vi "Bloch Sphere - Display.vi"(7 "QuWire in":refnum<class "QuWire.lvclass">) -> ()   [LabVIEW 2020]
uses:
  QuSim/QuWire/QuWire.lvclass
  <vilib>/Utility/miscctls.llb/LV3DPointTypeDef.ctl
  <vilib>/picture/3D Picture Control/NI_3D Picture Control.lvlib
panel:
  out "3D Picture":refnum<vi>(3d-picture)
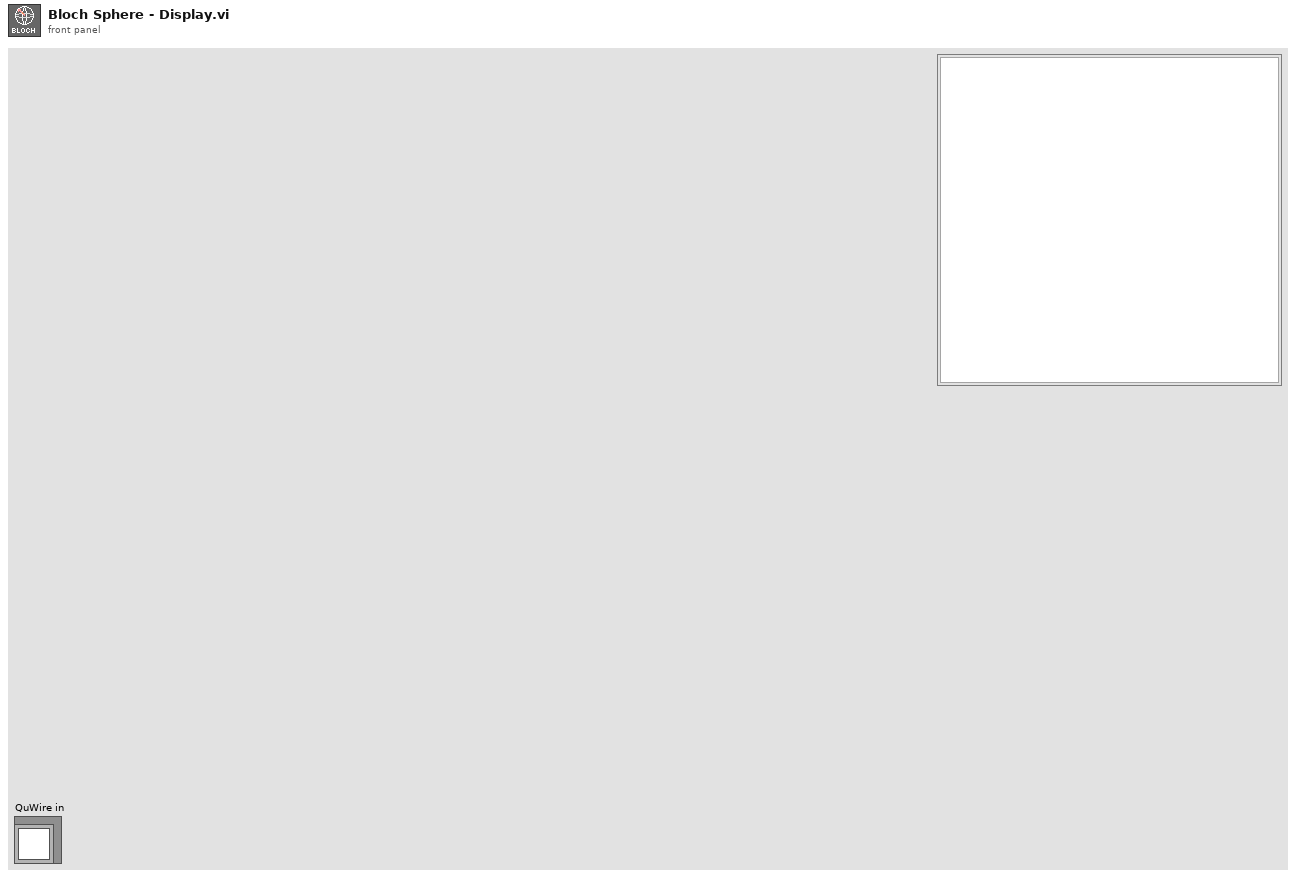
[diagram p1: front panel]
types:
  T1 = typedef "LV3DPointTypeDef.ctl" = cluster{"X":sgl, "Y":sgl, "Z":sgl}
  T2 = enum16{"None", "Spherical", "Flying", "Oriented"}
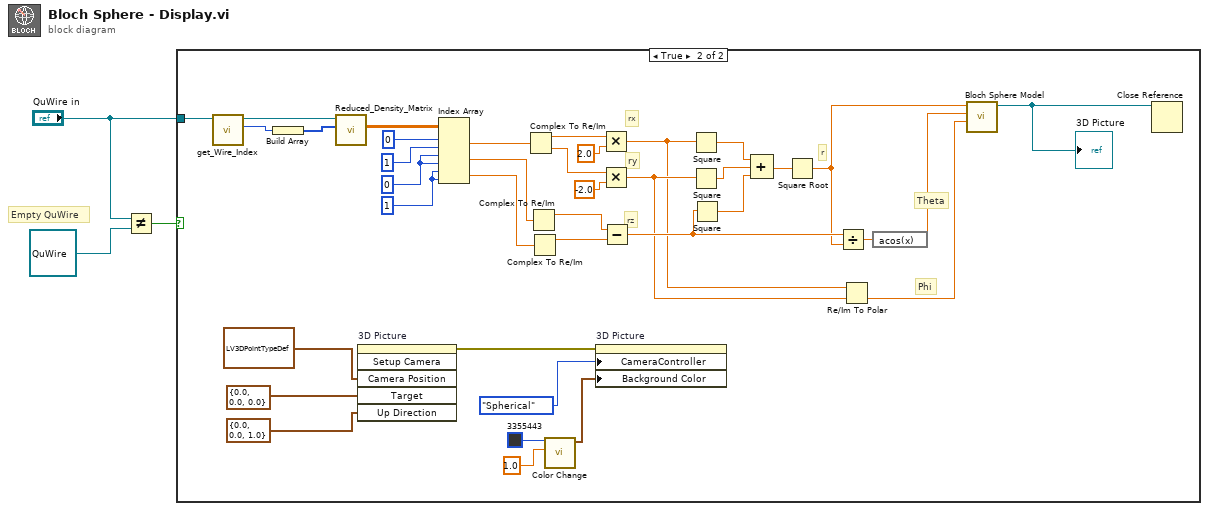
[diagram p0: block diagram]
diagram:
  # "Empty QuWire"
  n1 = Not Equal?(x="QuWire in", y=refnum<class "QuWire.lvclass"> refnum ("QuWire in")) -> (x != y?=w2:bool)
  n2 = case shown="True" w2 {
    tunnel: "QuWire in" -> [_ w18]
    frame False {
    }
    frame True {
      w38 = 1 ("disabled index (col)")
      w39 = 0 ("index (row)")
      # "Phi"
      # "Theta"
      # "r"
      # "rz"
      # "ry"
      # "rx"
      n3 = call "get_Wire_Index.vi"("QuWire in"=w18) -> ("Wire Index"=w16:i32, "QuWire out"=w17:refnum<class "QuWire.lvclass">)  [unwired: 8 in, 1 out]
      n4 = Build Array(w16) -> (w20:i32[])
      n5 = call "Reduced_Density_Matrix.vi"("Qubits to Keep"=w20, "QuWire in"=w17) -> ("Reduced Density Matrix"=w19:cdb[][])  [unwired: 6 in, 3 out]
      n6 = invoke on="3D Picture" class="SceneGraphDisp (strict)" method="Setup Camera"("Camera Position"=T1 {"X"=2.4, "Y"=1.6, "Z"=1.6}, "Target"=T1 {"X"=0.0, "Y"=0.0, "Z"=0.0}, "Up Direction"=T1 {"X"=0.0, "Y"=0.0, "Z"=1.0}) -> (error out=w8:errorcluster)  [unwired: 3 in, 5 out]
      n7 = Index Array(array=w19, index (row) #1=0 ("index (row)"), index (col) #1=1 ("disabled index (col)"), index (row) #2=w39, index (col) #2=w39, index (row) #3=w38, index (col) #3=w38) -> (element #1=w37:cdb, element #2=w31:cdb, element #3=w30:cdb)
      n8 = Complex To Re/Im(x + iy=w37) -> (x=w36:dbl, y=w33:dbl)
      n9 = Complex To Re/Im(x + iy=w31) -> (x=w28:dbl)  [unwired: 1 out]
      n10 = Complex To Re/Im(x + iy=w30) -> (x=w29:dbl)  [unwired: 1 out]
      n11 = call <vilib>:"Color Change.vi"("Alpha"=1.0, "Color"=u32 3355443 ("BG Color")) -> ("RGBA"=w7:cluster{"R":sgl, "G":sgl, "B":sgl, "A":sgl})  [unwired: 9 in]
      n12 = property on="3D Picture" class="SceneGraphDisp (strict)"(error in=w8, "CameraController"=T2."Spherical" ("Camera Controller:Type"), "Background Color"=w7) -> ()  [unwired: 1 in, 2 out]
      n13 = Multiply(x=w36, y=2.0) -> (x*y=w21:dbl)
      n14 = Multiply(x=w33, y=-2.0) -> (x*y=w22:dbl)
      n15 = Subtract(x=w28, y=w29) -> (x-y=w26:dbl)
      n16 = Square(x=w21) -> (x^2=w24:dbl)
      n17 = Square(x=w22) -> (x^2=w23:dbl)
      n18 = Square(x=w26) -> (x^2=w32:dbl)
      n19 = Compound Arithmetic op=ADD(w24, w23, w32) -> (w27:dbl)
      n20 = Square Root(x=w27) -> (sqrt(x)=w14:dbl)
      n21 = Divide(x=w26, y=w14) -> (x/y=w25:dbl)
      n22 = Re/Im To Polar(2:w22, 3:w21) -> (0:w12:dbl)  [unwired: 1 out]
      n23 = expression code="acos(x)"(w25) -> (w13:dbl)
      n24 = call "Bloch Sphere Model.vi"("Phi"=w12, "Theta"=w13, "Length"=w14) -> ("SceneObject out"=w15:refnum<vi>)  [unwired: 8 in]
      "3D Picture" <- w15
      n25 = Close Reference(reference=w15) -> ()  [unwired: 1 in, 1 out]
    }
  }
